vi "Shutdown.vi"(8 "error in (no error)":errorcluster, 10 "Reply Channel":refnum<notifier>, 11 "Dev View in":refnum<class "Dev View.lvclass">) -> (0 "error out":errorcluster, 3 "Dev View out":refnum<class "Dev View.lvclass">)   [LabVIEW 2015, in "Dev View.lvclass"]
uses:
  Dev View.lvclass
  Re-use Libraries/Minimal Actor Framework/Messaging/Message/Message.lvclass
  Re-use Libraries/Minimal Actor Framework/Actors/Base Actor/Actor/Actor.lvclass
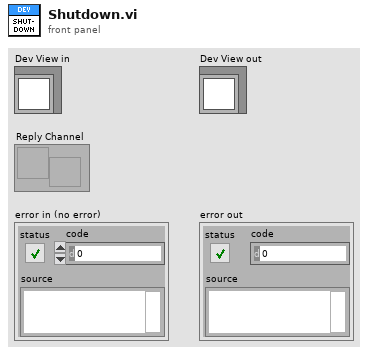
[diagram p1: front panel]
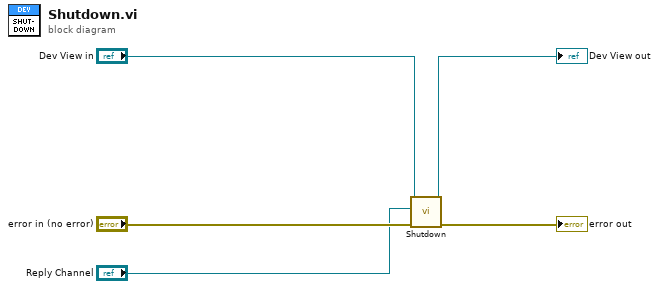
[diagram p0: block diagram]
diagram:
  n1 = call-parent "Shutdown.vi"("error in (no error)"="error in (no error)", "Reply Channel"="Reply Channel", "Actor in"="Dev View in") -> ("error out"=→"error out":errorcluster, "Actor out"=→"Dev View out":refnum<class "Dev View.lvclass">)  [unwired: 7 in]
